vi "ctrlManualThrustersHost.vi"() -> ()   [LabVIEW 2014]
panel:
  in  "Switch to Dashboard":bool
  in  "Thruster pos 2":dbl(knob) min=-1.0 max=1.0 scale=-1.0..1.0
  in  "Power 2":dbl(slide) min=-1.0 max=1.0 scale=-1.0..1.0
  in  "Thruster pos 1":dbl(knob) min=-1.0 max=1.0 scale=-1.0..1.0
  in  "Power 1":dbl(slide) min=-1.0 max=1.0 scale=-1.0..1.0
  in  "Stop":bool
  in  "Thruster pos 0":dbl(knob) min=-1.0 max=1.0 scale=-1.0..1.0
  in  "Power 0":dbl(slide) min=-1.0 max=1.0 scale=-1.0..1.0
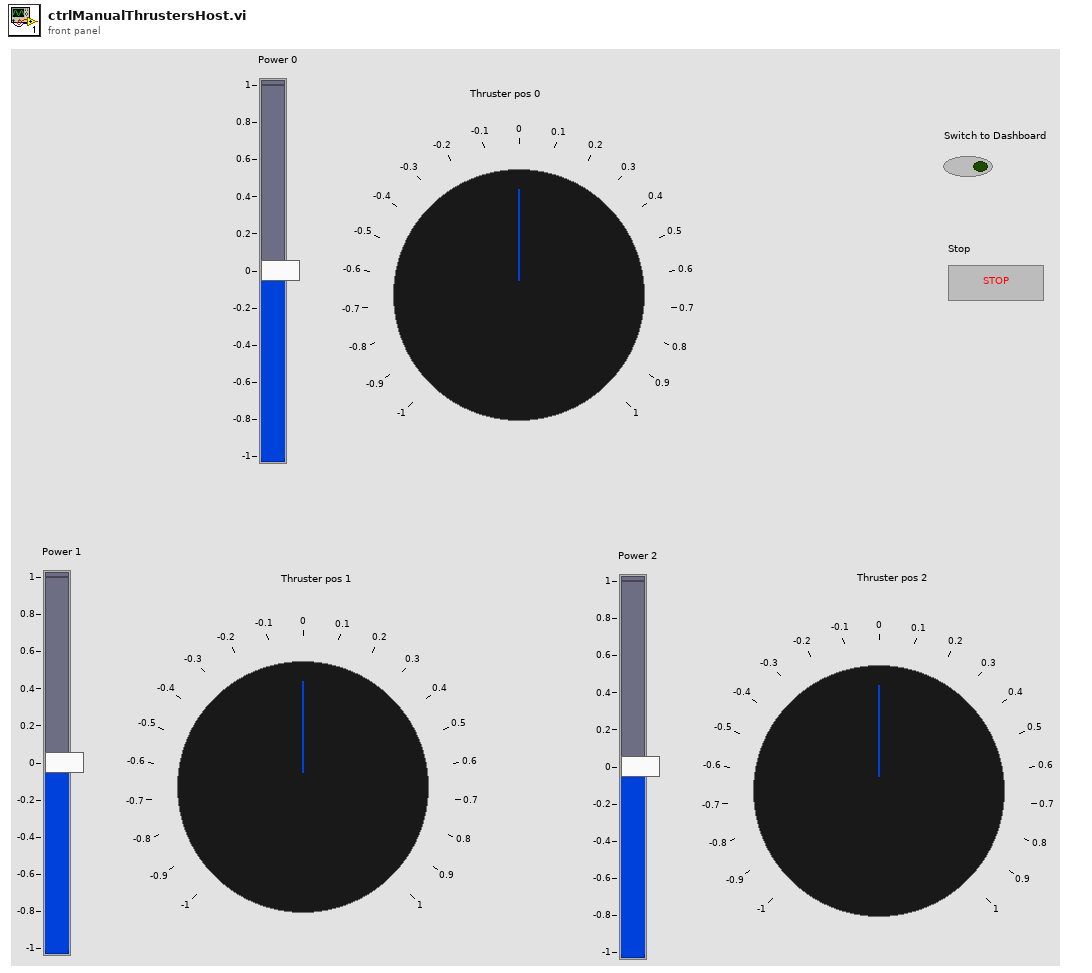
[diagram p1: front panel]
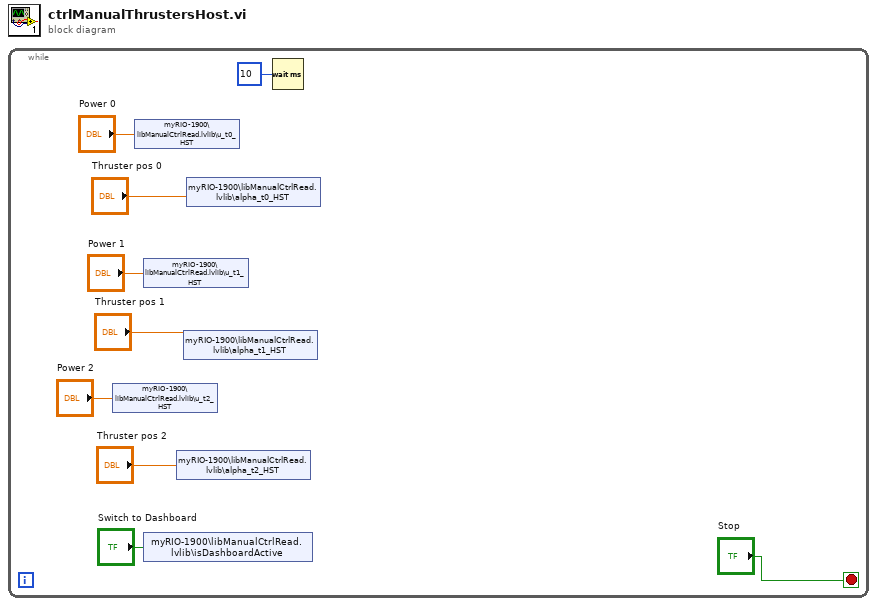
[diagram p0: block diagram]
diagram:
  n1 = while {
    stop <- "Stop" stop-if-true
    n2 = shared-variable "myRIO-1900\\libManualCtrlRead.lvlib\\u_t2_HST"("Power 2") -> ()  [unwired: 1 in, 1 out]
    n3 = shared-variable "myRIO-1900\\libManualCtrlRead.lvlib\\u_t0_HST"("Power 0") -> ()  [unwired: 1 in, 1 out]
    n4 = shared-variable "myRIO-1900\\libManualCtrlRead.lvlib\\u_t1_HST"("Power 1") -> ()  [unwired: 1 in, 1 out]
    n5 = shared-variable "myRIO-1900\\libManualCtrlRead.lvlib\\isDashboardActive"("Switch to Dashboard") -> ()  [unwired: 1 in, 1 out]
    n6 = shared-variable "myRIO-1900\\libManualCtrlRead.lvlib\\alpha_t2_HST"("Thruster pos 2") -> ()  [unwired: 1 in, 1 out]
    n7 = shared-variable "myRIO-1900\\libManualCtrlRead.lvlib\\alpha_t1_HST"("Thruster pos 1") -> ()  [unwired: 1 in, 1 out]
    n8 = shared-variable "myRIO-1900\\libManualCtrlRead.lvlib\\alpha_t0_HST"("Thruster pos 0") -> ()  [unwired: 1 in, 1 out]
    n9 = Wait (ms)(milliseconds to wait=u32 10) -> ()  [unwired: 1 out]
  }
